vi "Destroy Events Refs.vi"(11 "Event Actor in":refnum<class "Event Actor.lvclass">) -> (3 "Event Actor out":refnum<class "Event Actor.lvclass">)   [LabVIEW 2021, in "jettl.lvlib" / "Event Actor.lvclass"]
uses:
  Event Actor.lvclass
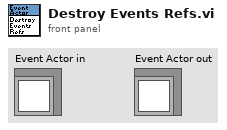
[diagram p1: front panel]
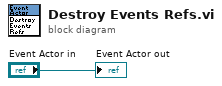
[diagram p0: block diagram]
diagram:
  "Event Actor out" <- "Event Actor in"
